vi "storelist输出.vi"(9 "CM":i32, 10 "storelist":string, 11 "storelist":string[][](array[string])) -> (3 "输出数组":string[][](array[string]))   [LabVIEW 2014]
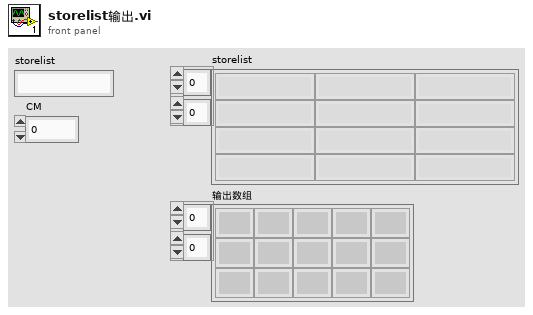
[diagram p1: front panel]
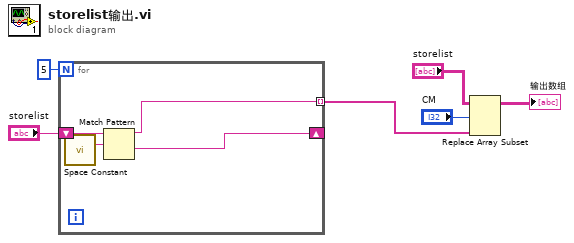
[diagram p0: block diagram]
diagram:
  n1 = for {
    N: 5 -> [_]
    shift-right: [w9] -> _
    shift-left: "storelist" -> [w10]
    tunnel: [w8] -> w3 mode=indexing
    n2 = call <vilib>:"Space Constant.vi"() -> ("String"=w7:string)
    n3 = Match Pattern(string=w10, regular expression=w7) -> (before substring=w8:string, after substring=w9:string)  [unwired: 1 in, 2 out]
  }
  n4 = Replace Array Subset(array="storelist", new element=w3, index (row)="CM") -> (→"输出数组":string[][])  [unwired: 1 in]
